vi "lpf3.vi"(8 "filter_gain":dbl=0.000627923994, 10 "In1":dbl) -> (2 "Out1":dbl)   [LabVIEW 2012]
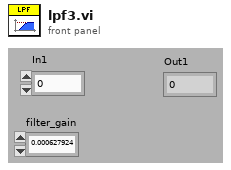
[diagram p1: front panel]
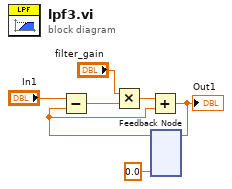
[diagram p0: block diagram]
diagram:
  n1 = feedback #1(0.0) -> (w4:dbl)
  n2 = Subtract(x="In1", y=w4) -> (x-y=w6:dbl)
  n3 = Multiply(x="filter_gain", y=w6) -> (x*y=w2:dbl)
  n4 = Add(x=w2, y=w4) -> (x+y=w3:dbl)
  "Out1" <- w3
  n5 = feedback-in #1(w3) -> ()
